vi "PlotTve.vi"(7 "Clear? (f)":bool, 8 "error in (no error)":errorcluster, 11 "Data real time":dbl[](array[numeric])) -> (0 "error out":errorcluster, 3 "TVE":cluster{timestamp[], dbl[]}[](graph))   [LabVIEW 2018, in "Visualization.lvlib" / "VisualizeAnalysis.lvclass"]
uses:
  VisualizeAnalysis.lvclass
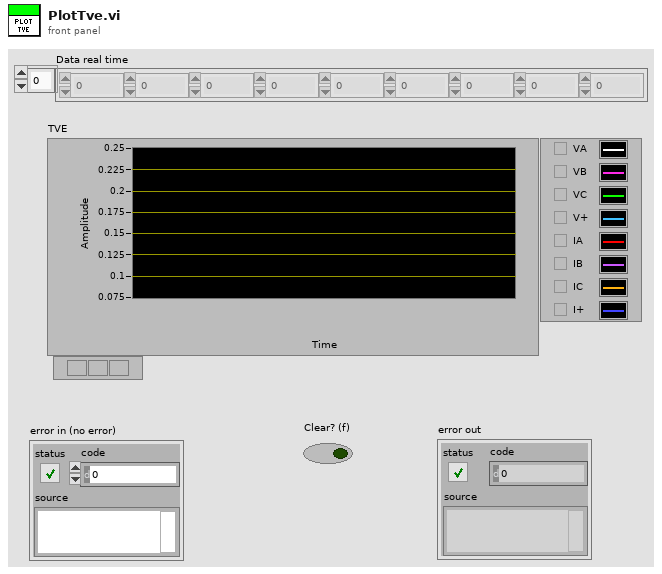
[diagram p1: front panel]
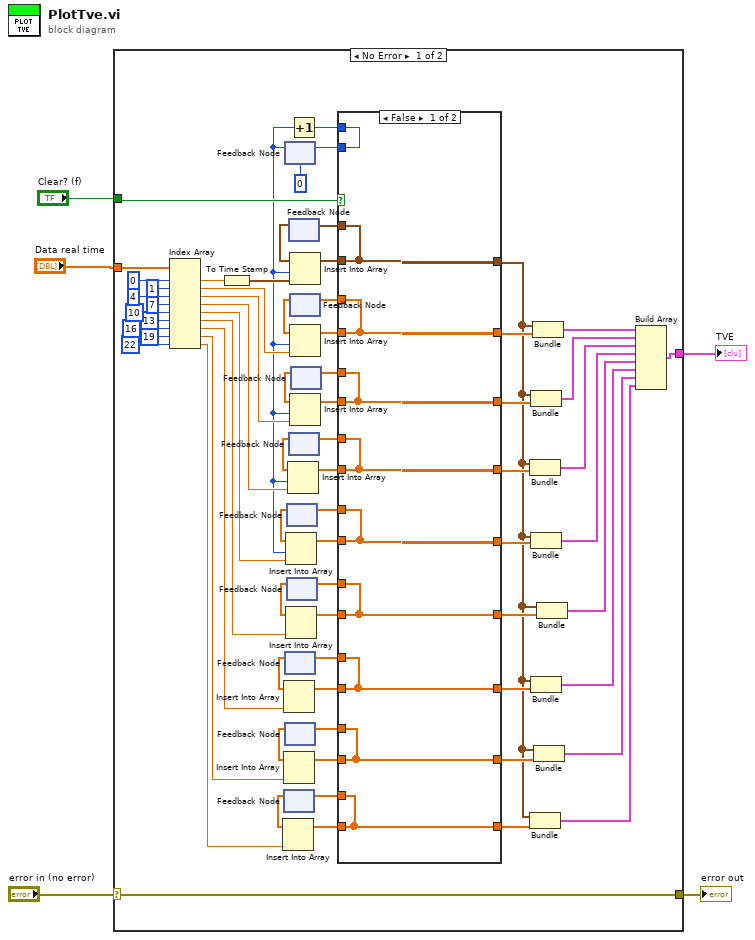
[diagram p0: block diagram]
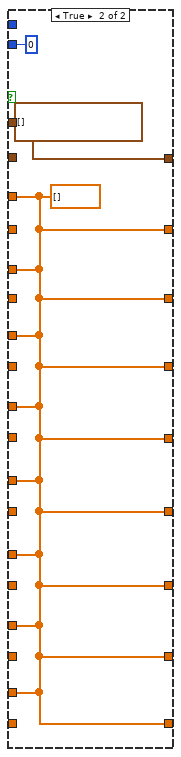
[diagram p2: hidden frame]
diagram:
  n1 = case shown="No Error" "error in (no error)" {
    selector: "error in (no error)" -> [w35 w90]
    tunnel: "Clear? (f)" -> [w76 _]
    tunnel: "Data real time" -> [w75 _]
    tunnel: [w65 _] -> w3
    tunnel: [w35 w90] -> w1
    frame No Error {
      n2 = Index Array(array=w75, index #1=0 ("index"), index #2=1 ("index"), index #3=4 ("index"), index #4=7 ("index"), index #5=10 ("index"), index #6=13 ("index"), index #7=16 ("index"), index #8=19 ("index"), index #9=22 ("index")) -> (element #1=w64:dbl, element #2=w73:dbl, element #3=w72:dbl, element #4=w71:dbl, element #5=w70:dbl, element #6=w29:dbl, element #7=w28:dbl, element #8=w27:dbl, element #9=w12:dbl)
      n3 = To Time Stamp(1:w64) -> (0:w74:timestamp)
      n4 = feedback #1() -> (w6:dbl[])  [unwired: 1 in]
      n5 = Insert Into Array(array=w6, new element=w12) -> (w11:dbl[])  [unwired: 1 in]
      n6 = feedback #2(u32 0) -> (w58:u32)
      n7 = feedback #3() -> (w15:dbl[])  [unwired: 1 in]
      n8 = Insert Into Array(array=w15, new element=w28) -> (w26:dbl[])  [unwired: 1 in]
      n9 = feedback #4() -> (w14:dbl[])  [unwired: 1 in]
      n10 = Insert Into Array(array=w14, new element=w27) -> (w25:dbl[])  [unwired: 1 in]
      n11 = feedback #5() -> (w57:dbl[])  [unwired: 1 in]
      n12 = Insert Into Array(array=w57, index=w58, new element=w70) -> (w55:dbl[])
      n13 = feedback #6() -> (w16:dbl[])  [unwired: 1 in]
      n14 = Insert Into Array(array=w16, new element=w29) -> (w31:dbl[])  [unwired: 1 in]
      n15 = Increment(x=w58) -> (x+1=w44:u32)
      n16 = feedback #7() -> (w40:timestamp[])  [unwired: 1 in]
      n17 = feedback #8() -> (w54:dbl[])  [unwired: 1 in]
      n18 = Insert Into Array(array=w54, index=w58, new element=w71) -> (w52:dbl[])
      n19 = Insert Into Array(array=w40, index=w58, new element=w74) -> (w41:timestamp[])
      n20 = feedback #9() -> (w48:dbl[])  [unwired: 1 in]
      n21 = Insert Into Array(array=w48, index=w58, new element=w73) -> (w46:dbl[])
      n22 = feedback #10() -> (w51:dbl[])  [unwired: 1 in]
      n23 = Insert Into Array(array=w51, index=w58, new element=w72) -> (w49:dbl[])
      n24 = case shown="False" w76 {
        tunnel: w41 -> [w85 _]
        tunnel: [w85 w88] -> w42
        tunnel: w44 -> [w86 _]
        tunnel: [w86 u32 0] -> w45
        tunnel: [w85 w88] -> w9
        tunnel: w46 -> [w84 _]
        tunnel: [w84 w87] -> w47
        tunnel: [w84 w87] -> w69
        tunnel: w49 -> [w83 _]
        tunnel: [w83 w87] -> w50
        tunnel: [w83 w87] -> w68
        tunnel: w52 -> [w82 _]
        tunnel: [w82 w87] -> w53
        tunnel: w55 -> [w81 _]
        tunnel: [w81 w87] -> w56
        tunnel: [w82 w87] -> w67
        tunnel: [w81 w87] -> w66
        tunnel: w31 -> [w80 _]
        tunnel: [w80 w87] -> w30
        tunnel: [w79 w87] -> w24
        tunnel: w26 -> [w79 _]
        tunnel: [w78 w87] -> w23
        tunnel: w25 -> [w78 _]
        tunnel: [w80 w87] -> w19
        tunnel: [w79 w87] -> w18
        tunnel: [w78 w87] -> w17
        tunnel: [w77 w87] -> w10
        tunnel: w11 -> [w77 _]
        tunnel: [w77 w87] -> w7
        frame False {
        }
        frame True {
          w87 = dbl[] []
          w88 = timestamp[] []
        }
      }
      n25 = feedback-in #1(w7) -> ()
      n26 = feedback-in #2(w45) -> ()
      n27 = feedback-in #3(w18) -> ()
      n28 = feedback-in #4(w17) -> ()
      n29 = feedback-in #5(w56) -> ()
      n30 = feedback-in #6(w19) -> ()
      n31 = feedback-in #7(w42) -> ()
      n32 = feedback-in #8(w53) -> ()
      n33 = feedback-in #9(w47) -> ()
      n34 = feedback-in #10(w50) -> ()
      n35 = Bundle(w9, w67) -> (w37:cluster{timestamp[], dbl[]})  [unwired: 1 in]
      n36 = Bundle(w9, w10) -> (w8:cluster{timestamp[], dbl[]})  [unwired: 1 in]
      n37 = Bundle(w9, w68) -> (w38:cluster{timestamp[], dbl[]})  [unwired: 1 in]
      n38 = Bundle(w9, w66) -> (w36:cluster{timestamp[], dbl[]})  [unwired: 1 in]
      n39 = Bundle(w9, w24) -> (w21:cluster{timestamp[], dbl[]})  [unwired: 1 in]
      n40 = Bundle(w9, w69) -> (w39:cluster{timestamp[], dbl[]})  [unwired: 1 in]
      n41 = Bundle(w9, w23) -> (w20:cluster{timestamp[], dbl[]})  [unwired: 1 in]
      n42 = Bundle(w9, w30) -> (w22:cluster{timestamp[], dbl[]})  [unwired: 1 in]
      n43 = Build Array(w39, w38, w37, w36, w22, w21, w20, w8) -> (w65:cluster{timestamp[], dbl[]}[])
    }
    frame Error {
    }
  }
  "error out" <- w1
  "TVE" <- w3
